vi "PH_IEEE1394Camera.PC Write PSDB.vi"(0 "i ref in":refnum<vi>, 5 "error IO":errorcluster) -> (14 "i ref out":refnum<vi>, 19 "error out":errorcluster)   [LabVIEW 2014, in "PH_IEEE1394Camera.lvlib"]
doc: "This is the proc case which writes data to the PHELIX shot data base."
uses:
  PH_IEEE1394Camera.lvlib
  PH_Basics/PH_PSDBWriter/PH_PSDBWriter.lvlib
  PH_Basics/PH_Cam_BaseClass/PH_Cam_BaseClass.lvlib
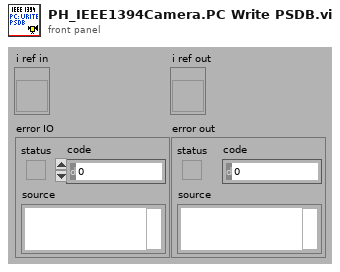
[diagram p1: front panel]
types:
  T1 = typedef "PH_IEEE1394Camera.lvlib/PH_IEEE1394Camera.i attribute.ctl" = cluster{"Gui Refs":cluster{"Brightness":refnum<vi>, "Shutter":refnum<vi>, "Gain":refnum<vi>, "Center of Gravity":refnum<vi>, "Supported Video Modes":refnum<vi>, "Trigger Polarity":refnum<vi>, "Trigger Mode":refnum<vi>, "Trigger Timeout":refnum<vi>, "Bit Depth":refnum<vi>, "Video Mode":refnum<vi>, "Top":refnum<vi>, "Bottom":refnum<vi>, "Left":refnum<vi>, "Right":refnum<vi>, "Set ROI to Maximum":refnum<vi>, "Camera Details":refnum<vi>, "Current Cam Attributes":refnum<vi>, "Attribute to set":refnum<vi>, "Num Value":refnum<vi>, "String Value":refnum<vi>, "Bool Value":refnum<vi>, "Set Cam Attribute":refnum<vi>}, "Cam":cluster{"IMAQ1394 Session":T2, "Camera Details":T3}, "Current Attributes":T4[], "Supported Video Modes ":cluster{"Video Mode":u32, "Video Mode Name":string}[], "Wanted Attributes":cluster{"Name":string, "Num Value":dbl, "String Value":string, "Boolean Value":bool}[], "Cam Attributes":T6}
  T2 = typedef "IMAQdx.ctl" = refnum<k21>
  T3 = typedef "PH_IEEE1394Camera.lvlib/PH_IEEE1394Camera.Cam Details.ctl" = cluster{"Model":string, "Serial Number":dbl, "Cam name (Machinery)":string, "Bus Type":string}
  T4 = typedef "PH_IEEE1394Camera.lvlib/PH_IEEE1394Camera.Cam Attribute.ctl" = cluster{"Information":cluster{"Type":T5, "Readable":bool, "Writable":bool, "Name":string}, "Num Value":dbl, "String Value":string, "Maximum":dbl, "Minimum":dbl, "Units":string, "Description":string, "EnumStrings[]":string[], "EnumValues[]":u32[], "Boolean Value":bool}
  T5 = typedef "NI_Vision_Acquisition_Software.lvlib/IMAQdx Attribute Type.ctl" = enum32{"U32", "I64", "DBL", "String", "Enum", "Bool", "Command"}
  T6 = typedef "PH_IEEE1394Camera.lvlib/PH_IEEE1394Camera.Relevant Cam Attributes.ctl" = cluster{"Video Mode":cluster{"Name":string, "Index":i32}, "Brightness":cluster{"Name":string, "Index":i32}, "Gain":cluster{"Name":string, "Index":i32}, "Shutter":cluster{"Name":string, "Index":i32}, "Trigger Pol":cluster{"Name":string, "Index":i32}, "Trigger Mode":cluster{"Name":string, "Index":i32}, "Timeout":cluster{"Name":string, "Index":i32}, "Bit Depth":cluster{"Name":string, "Index":i32}, "Pixel Bits":cluster{"Name":string, "Index":i32}, "Pixel Bytes":cluster{"Name":string, "Index":i32}, "Left":cluster{"Name":string, "Index":i32}, "Right":cluster{"Name":string, "Index":i32}, "Top":cluster{"Name":string, "Index":i32}, "Bottom":cluster{"Name":string, "Index":i32}}
  T7 = cluster{"Video Mode":u32, "Video Mode Name":string}[]
  T8 = cluster{"Video Mode":u32, "Video Mode Name":string}
  T9 = typedef "PH_PSDBWriter.lvlib/PH_PSDBWriter.Image dataset.ctl" = cluster{"name":string, "data":T10, "unit":string}
  T10 = typedef "IMAQ Image.ctl" = refnum<image>
  T11 = typedef "PH_PSDBWriter.lvlib/PH_PSDBWriter.String dataset.ctl" = cluster{"name":string, "data":string, "unit":string}
  T12 = typedef "PH_PSDBWriter.lvlib/PH_PSDBWriter.Boolean dataset.ctl" = cluster{"name":string, "data":bool, "unit":string}
  T13 = typedef "PH_PSDBWriter.lvlib/PH_PSDBWriter.Numeric dataset.ctl" = cluster{"name":string, "data":dbl, "unit":string}
  T14 = typedef "PH_PSDBWriter.lvlib/PH_PSDBWriter.PSDB Dataset.ctl" = cluster{"Version":i32, "2D data Input":T15[], "Boolean Input":T12[], "Image Input":T9[], "Numeric Input":T13[], "String Input":T11[]}
  T15 = typedef "PH_PSDBWriter.lvlib/PH_PSDBWriter.2D dataset.ctl" = cluster{"name":string, "data":dbl[][], "axis description":T16}
  T16 = typedef "PSDB.lvlib/PSDB_AxisDescription.ctl" = cluster{"x axis label":string, "y axis label":string, "x axis unit":string, "y axis unit":string}
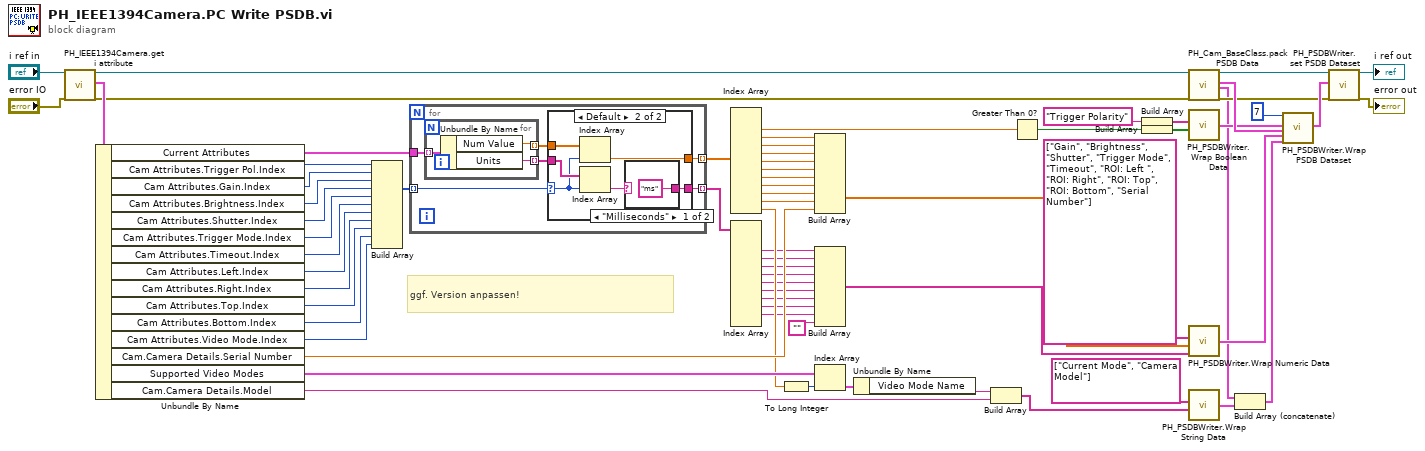
[diagram p0: block diagram]
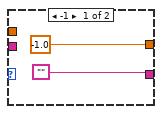
[diagram p2: hidden frame]
diagram:
  # "ggf. Version anpassen!"
  n1 = call "PH_IEEE1394Camera.get i attribute.vi"("i ref in"="i ref in", "error in (no error)"="error IO") -> ("i ref out"=w2:refnum<vi>, "i attribute"=w47:T1, "error out"=w1:errorcluster)  [unwired: 15 in]
  n2 = Unbundle By Name(w47) -> ("Current Attributes"=w46:T4[], "Cam Attributes.Trigger Pol.Index"=w45:i32, "Cam Attributes.Gain.Index"=w44:i32, "Cam Attributes.Brightness.Index"=w43:i32, "Cam Attributes.Shutter.Index"=w42:i32, "Cam Attributes.Trigger Mode.Index"=w41:i32, "Cam Attributes.Timeout.Index"=w40:i32, "Cam Attributes.Left.Index"=w33:i32, "Cam Attributes.Right.Index"=w32:i32, "Cam Attributes.Top.Index"=w31:i32, "Cam Attributes.Bottom.Index"=w30:i32, "Cam Attributes.Video Mode.Index"=w29:i32, "Cam.Camera Details.Serial Number"=w37:dbl, "Supported Video Modes"=w36:T7, "Cam.Camera Details.Model"=w35:string)
  n3 = Build Array(w45, w44, w43, w42, w41, w40, w33, w32, w31, w30, w29) -> (w39:i32[])
  n4 = for {
    tunnel: w46 -> [w74]
    tunnel: w39 -> [w69] mode=indexing
    tunnel: [w71] -> w28 mode=indexing
    tunnel: [w70] -> w16 mode=indexing
    n5 = for {
      tunnel: w74 -> [w87] mode=indexing
      tunnel: [w86] -> w73 mode=indexing
      tunnel: [w85] -> w72 mode=indexing
      n6 = Unbundle By Name(w87) -> ("Num Value"=w85:dbl, "Units"=w86:string)
    }
    n7 = case shown="Default" w69 {
      selector: w69 -> [_ w80]
      tunnel: w73 -> [_ w81]
      tunnel: w72 -> [_ w82]
      tunnel: ["" w77] -> w70
      tunnel: [-1.0 ("Num Value") w79] -> w71
      frame -1 {
      }
      frame Default {
        n8 = Index Array(array=w82, index=w80) -> (element=w79:dbl)
        n9 = Index Array(array=w81, index=w80) -> (element=w78:string)
        n10 = case shown="\"Milliseconds\"" w78 {
          selector: w78 -> [_ w84]
          tunnel: ["ms" w84] -> w77
          frame "Milliseconds" {
          }
          frame Default {
          }
        }
      }
    }
  }
  n11 = Index Array(array=w28) -> (element #1=w27:dbl, element #2=w26:dbl, element #3=w25:dbl, element #4=w24:dbl, element #5=w23:dbl, element #6=w22:dbl, element #7=w21:dbl, element #8=w20:dbl, element #9=w19:dbl, element #10=w18:dbl, element #11=w17:dbl)  [unwired: 11 in]
  n12 = Index Array(array=w16) -> (element #2=w14:string, element #3=w13:string, element #4=w12:string, element #5=w11:string, element #6=w10:string, element #7=w9:string, element #8=w8:string, element #9=w7:string, element #10=w6:string)  [unwired: 11 in, 2 out]
  n13 = To Long Integer(number=w17) -> (32bit integer=w38:i32)
  n14 = Build Array(w26, w25, w24, w23, w22, w21, w20, w19, w18, w37) -> (w15:dbl[])
  n15 = Build Array(w14, w13, w12, w11, w10, w9, w8, w7, w6, "") -> (w34:string[])
  n16 = Index Array(array=w36, index=w38) -> (element=w66:T8)
  n17 = Unbundle By Name(w66) -> ("Video Mode Name"=w48:string)
  n18 = Build Array(w48, w35) -> (w63:string[])
  n19 = Greater Than 0?(x=w27) -> (x > 0?=w54:bool)
  n20 = Build Array("Trigger Polarity" ("name")) -> (w51:string[])
  n21 = Build Array(w54) -> (w52:bool[])
  n22 = call "PH_Cam_BaseClass.pack PSDB Data.vi"("VI in"=w2, "error in (no error)"=w1) -> ("VI out"=w49:refnum<vi>, "PSDB Image Data Array"=w57:T9[], "PSDB String Data Array"=w3:T11[], "error out"=w50:errorcluster)  [unwired: 14 in]
  n23 = call "PH_PSDBWriter.Wrap Boolean Data.vi"("Data Array"=w52, "Name Array"=w51) -> ("PSDB Boolean Data Array"=w56:T12[])  [unwired: 2 in]
  n24 = call "PH_PSDBWriter.Wrap Numeric Data.vi"("Unit Array"=w34, "Data Array"=w15, "Name Array"=string[] ["Gain", "Brightness", "Shutter", "Trigger Mode", "Timeout", "ROI: Left ", "ROI: Right", "ROI: Top", "ROI: Bottom", "Serial Number"]) -> ("PSDB Numeric Data Array"=w58:T13[])  [unwired: 1 in]
  n25 = call "PH_PSDBWriter.Wrap String Data.vi"("Data Array"=w63, "Name Array"=string[] ["Current Mode", "Camera Model"]) -> ("PSDB String Data Array"=w62:T11[])  [unwired: 2 in]
  n26 = Build Array (concatenate)(w3, w62) -> (w4:T11[])
  n27 = call "PH_PSDBWriter.Wrap PSDB Dataset.vi"("Version"=7, "Boolean Input"=w56, "Image Input"=w57, "Numeric Input"=w58, "String Input"=w4) -> ("PSDB Dataset"=w61:T14)  [unwired: 14 in]
  n28 = call "PH_PSDBWriter.set PSDB Dataset.vi"("VI in"=w49, "PSDB Dataset"=w61, "error in (no error)"=w50) -> ("VI out"=→"i ref out":refnum<vi>, "error out"=→"error out":errorcluster)  [unwired: 15 in]
